vi "Update GUI.vi"(8 "error in (no error)":errorcluster, 11 "ImageStack in":refnum<class "ImageStack.lvclass">) -> (0 "error out":errorcluster, 3 "ImageStack out":refnum<class "ImageStack.lvclass">)   [LabVIEW 2012, in "ImageStack.lvclass"]
uses:
  ImageStack.lvclass
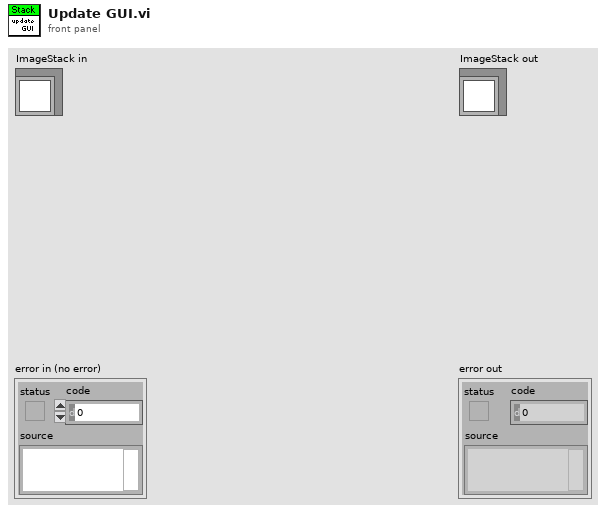
[diagram p1: front panel]
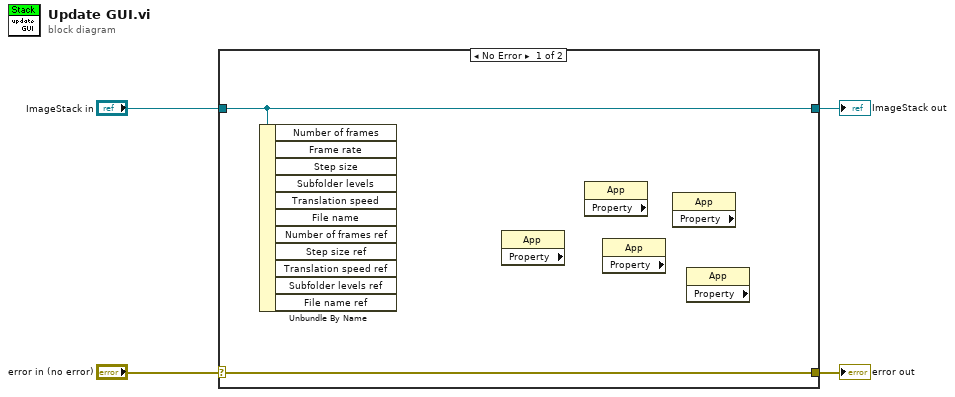
[diagram p0: block diagram]
diagram:
  n1 = case shown="No Error" "error in (no error)" {
    selector: "error in (no error)" -> [w6 w8]
    tunnel: [w6 w8] -> w3
    tunnel: [w5 w7] -> w1
    tunnel: "ImageStack in" -> [w5 w7]
    frame No Error {
      n2 = Unbundle By Name(w5) -> ()  [unwired: 11 out]
      n3 = property class="App" props=[]() -> ()  [unwired: 2 in, 3 out]
      n4 = property class="App" props=[]() -> ()  [unwired: 2 in, 3 out]
      n5 = property class="App" props=[]() -> ()  [unwired: 2 in, 3 out]
      n6 = property class="App" props=[]() -> ()  [unwired: 2 in, 3 out]
      n7 = property class="App" props=[]() -> ()  [unwired: 2 in, 3 out]
    }
    frame Error {
    }
  }
  "error out" <- w3
  "ImageStack out" <- w1
